vi "Inverse_Kinematics_noErrMsg_v2.vi"(4 "B3":dbl[](array[numeric]), 5 "px":dbl, 6 "pz":dbl, 7 "B2":dbl[](array[numeric]), 8 "py":dbl, 9 "B1":dbl[](array[numeric])) -> (1 "theta 3":dbl, 2 "theta 2":dbl, 3 "theta 1":dbl)   [LabVIEW 2016]
doc: "This VI converts the desired tool tip position (px,py,pz) into joint motions of theta 1, theta 2, and theta 3.\nB1, B2, and B3 are 2-element arrays containing lower and upper bounds for joint motions.\n\"Reset Inputs\" sends out a boolean value (T) if an error occurs."
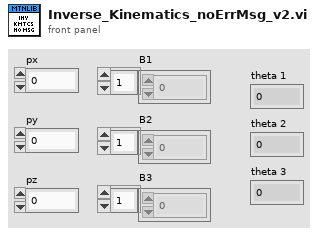
[diagram p1: front panel]
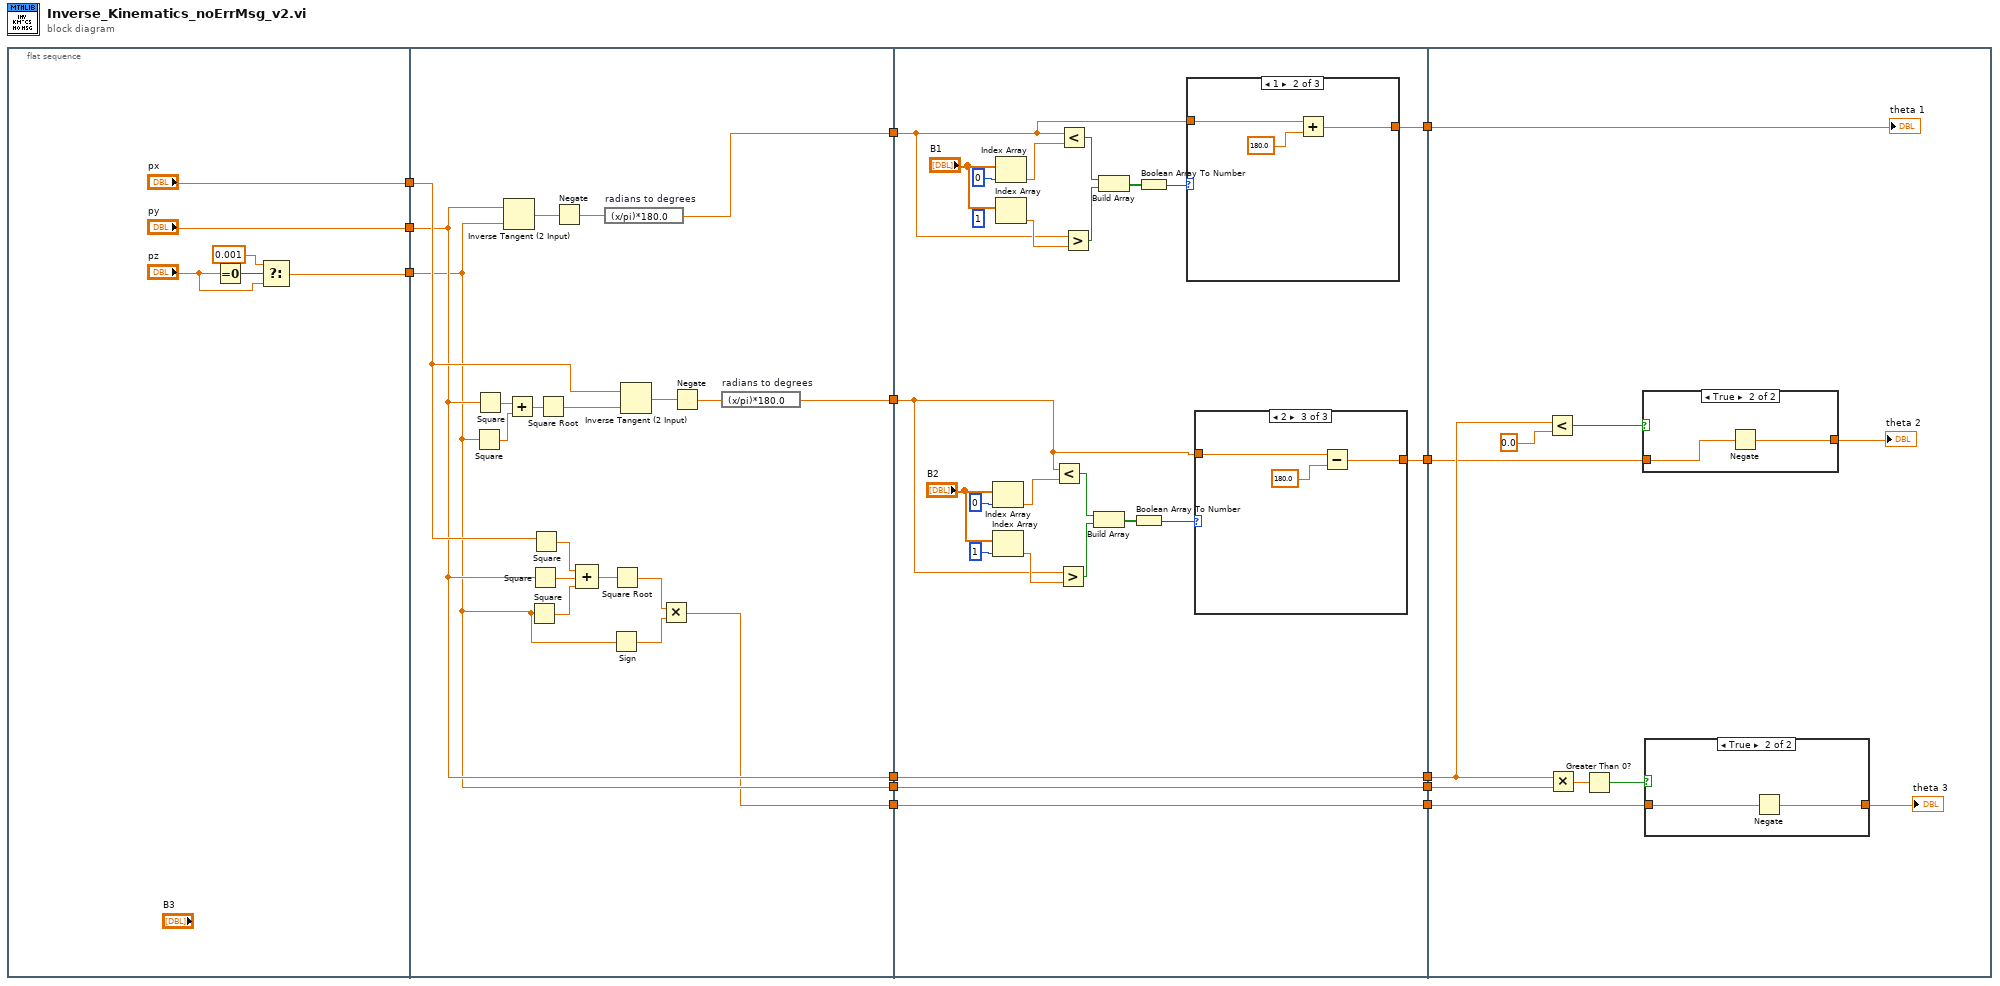
[diagram p0: block diagram]
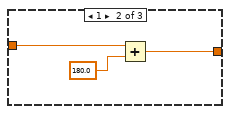
[diagram p3: hidden frame]
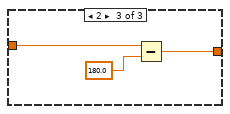
[diagram p5: hidden frame]
diagram:
  n1 = flat-sequence {
    tunnel: ["py"] -> w13
    tunnel: [w15] -> w12
    tunnel: ["px"] -> w11
    tunnel: w13 -> [w26]
    tunnel: w12 -> [w25]
    tunnel: w11 -> [w29]
    tunnel: [w28] -> w10
    tunnel: [w27] -> w9
    tunnel: [w26] -> w7
    tunnel: [w25] -> w5
    tunnel: [w24] -> w3
    tunnel: w10 -> [w55]
    tunnel: w9 -> [w45]
    tunnel: [w44] -> w8
    tunnel: w7 -> [w44]
    tunnel: [w43] -> w6
    tunnel: w5 -> [w43]
    tunnel: [w42] -> w4
    tunnel: w3 -> [w42]
    tunnel: [w41] -> w2
    tunnel: [w40] -> w1
    tunnel: w8 -> [w83]
    tunnel: w6 -> [w82]
    tunnel: w4 -> [w85]
    tunnel: w2 -> [w81]
    tunnel: w1 -> [w79]
    frame #0 {
      n2 = Equal To 0?(x="pz") -> (x = 0?=w17:bool)
      n3 = Select(t=0.001, s=w17, f="pz") -> (s? t:f=w15:dbl)
    }
    frame #1 {
      n4 = Square(x=w25) -> (x^2=w33:dbl)
      n5 = Square(x=w26) -> (x^2=w32:dbl)
      n6 = Inverse Tangent (2 Input)(1:w25, 2:w26) -> (0:w22:dbl)
      n7 = Add(x=w32, y=w33) -> (x+y=w34:dbl)
      n8 = Square(x=w25) -> (x^2=w38:dbl)
      n9 = Square(x=w26) -> (x^2=w37:dbl)
      n10 = Square(x=w29) -> (x^2=w36:dbl)
      n11 = Square Root(x=w34) -> (sqrt(x)=w35:dbl)
      n12 = Negate(x=w22) -> (-x=w23:dbl)
      n13 = Compound Arithmetic op=ADD(w36, w37, w38) -> (w39:dbl)
      n14 = expression code="(x/pi)*180.0" "radians to degrees"(w23) -> (w28:dbl)
      n15 = Sign(1:w25) -> (0:w30:dbl)
      n16 = Square Root(x=w39) -> (sqrt(x)=w31:dbl)
      n17 = Inverse Tangent (2 Input)(1:w35, 2:w29) -> (0:w21:dbl)
      n18 = Multiply(x=w31, y=w30) -> (x*y=w24:dbl)
      n19 = Negate(x=w21) -> (-x=w20:dbl)
      n20 = expression code="(x/pi)*180.0" "radians to degrees"(w20) -> (w27:dbl)
    }
    frame #2 {
      (unwired) 1 ("index")
      n21 = Index Array(array="B2", index=0) -> (element=w48:dbl)
      n22 = Index Array(array="B2", index=1) -> (element=w47:dbl)
      n23 = Index Array(array="B1", index=0) -> (element=w61:dbl)
      n24 = Index Array(array="B1") -> (element=w60:dbl)  [unwired: 1 in]
      n25 = Less?(x=w45, y=w48) -> (x < y?=w49:bool)
      n26 = Greater?(x=w45, y=w47) -> (0:w50:bool)
      n27 = Less?(x=w55, y=w61) -> (x < y?=w59:bool)
      n28 = Greater?(x=w55, y=w60) -> (0:w58:bool)
      n29 = Build Array(w49, w50) -> (w51:bool[])
      n30 = Build Array(w59, w58) -> (w57:bool[])
      n31 = Boolean Array To Number(Boolean array=w51) -> (number=w46:u32)
      n32 = Boolean Array To Number(Boolean array=w57) -> (number=w56:u32)
      n33 = case shown="1" w56 {
        tunnel: w55 -> [w71 w73 w76]
        tunnel: [w71 w72 w75] -> w41
        frame 0, Default {
        }
        frame 1 {
          n34 = Add(x=w73, y=180.0) -> (x+y=w72:dbl)
        }
        frame 2 {
          n35 = Subtract(x=w76, y=180.0) -> (x-y=w75:dbl)
        }
      }
      n36 = case shown="2" w46 {
        tunnel: w45 -> [w64 w66 w69]
        tunnel: [w64 w65 w68] -> w40
        frame 0, Default {
        }
        frame 1 {
          n37 = Add(x=w66, y=180.0) -> (x+y=w65:dbl)
        }
        frame 2 {
          n38 = Subtract(x=w69, y=180.0) -> (x-y=w68:dbl)
        }
      }
    }
    frame #3 {
      n39 = Less?(x=w83, y=0.0) -> (x < y?=w80:bool)
      n40 = Multiply(x=w83, y=w82) -> (x*y=w87:dbl)
      n41 = Greater Than 0?(x=w87) -> (x > 0?=w86:bool)
      n42 = case shown="True" w80 {
        tunnel: w79 -> [w92 w94]
        tunnel: [w92 w93] -> w78
        frame False {
        }
        frame True {
          n43 = Negate(x=w94) -> (-x=w93:dbl)
        }
      }
      "theta 2" <- w78
      n44 = case shown="True" w86 {
        tunnel: w85 -> [w89 w91]
        tunnel: [w89 w90] -> w84
        frame False {
        }
        frame True {
          n45 = Negate(x=w91) -> (-x=w90:dbl)
        }
      }
      "theta 3" <- w84
      "theta 1" <- w81
    }
  }
